vi "I32_to_um.vi"   [LabVIEW 2023]
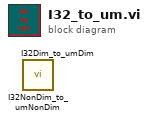
[diagram p0: block diagram]
diagram:
  n1 = call "I32NonDim_to_umNonDim.vi"() -> ()  [unwired: 11 in, 1 out]
  n2 = call "I32Dim_to_umDim.vi"() -> ()  [unwired: 11 in, 1 out]
